vi "GEvt-Generate State Change Log.vi"(0 "CSM Global Log Event":refnum<user-event>, 1 "Current State":string, 2 "Arguments":string, 3 "Source Message.*State":string, 4 "Source Message.*Arguments":string, 5 "Source Module":string, 6 "Name(\"\" to use uuid)":string, 10 "CSM:LogFilter.lvclass":refnum<class "LogFilter.lvclass">) -> (14 "CSM Global Log Event out":refnum<user-event>, 16 "event data":T1={"Name(\"\" to use uuid)"="", "Current State"="", "Arguments"="", "Source Message"={"‘State"="", "’Arguments"="", "’Error"={"status"=FALSE, "code"=0, "source"=""}}, "Source Module"="", "Complete(T)/Start(F)"=FALSE, "LogType"=enum."State Change"})   [LabVIEW 2020, in "Communicable State Machine.lvlib"]
uses:
  Communicable State Machine.lvlib
  _CSM_GlobalLog_MSG.ctl
  _CSM_Response Source Message.ctl
  _CSM_GlobalLog_MSG_TYPE.ctl
  LogFilter.lvclass
  Filter Check.vi
  Group Check - CSM.vi
  Group Check - LogType.vi
  Group Check - State.vi
  CSM Check - LogType.vi
  CSM Check - State.vi
  CSM Check - StateType.vi
  Group Check - StateType.vi
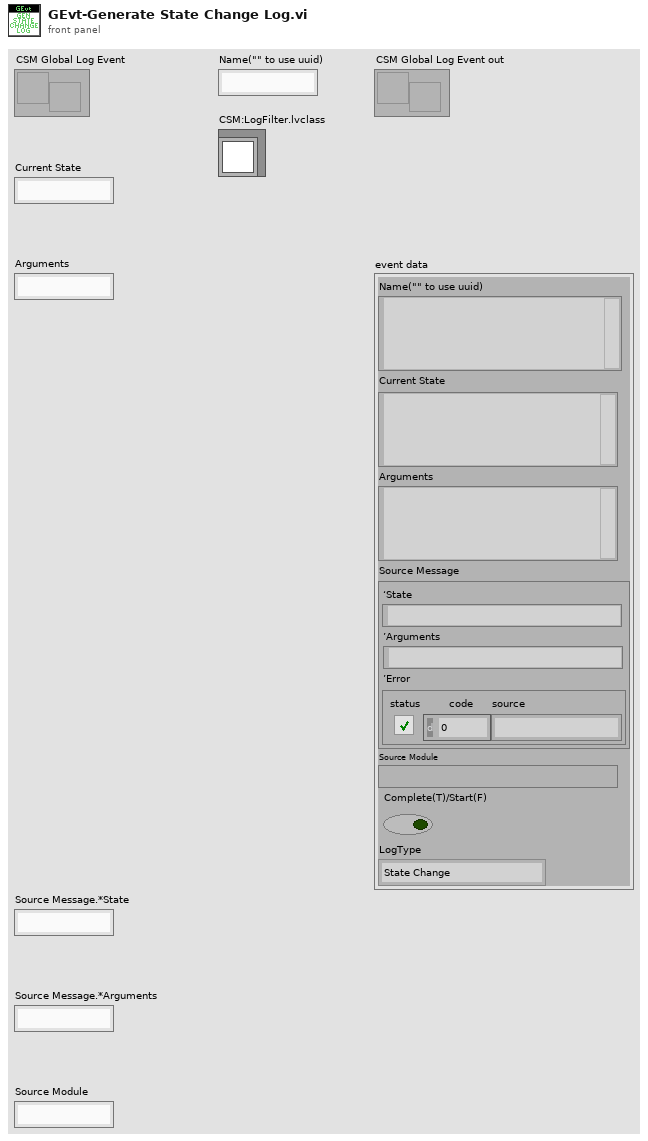
[diagram p1: front panel]
types:
  T1 = typedef "Communicable State Machine.lvlib/_CSM_GlobalLog_MSG.ctl" = cluster{"Name(\"\" to use uuid)":string, "Current State":string, "Arguments":string, "Source Message":T2, "Source Module":string, "Complete(T)/Start(F)":bool, "LogType":T3}
  T2 = typedef "Communicable State Machine.lvlib/_CSM_Response Source Message.ctl" = cluster{"‘State":string, "’Arguments":string, "’Error":errorcluster}
  T3 = typedef "Communicable State Machine.lvlib/_CSM_GlobalLog_MSG_TYPE.ctl" = enum16{"User Log", "State Change", "Status", "Interrupt", "Register", "Unregister", "Error Log", "Module Created", "Module Destroyed"}
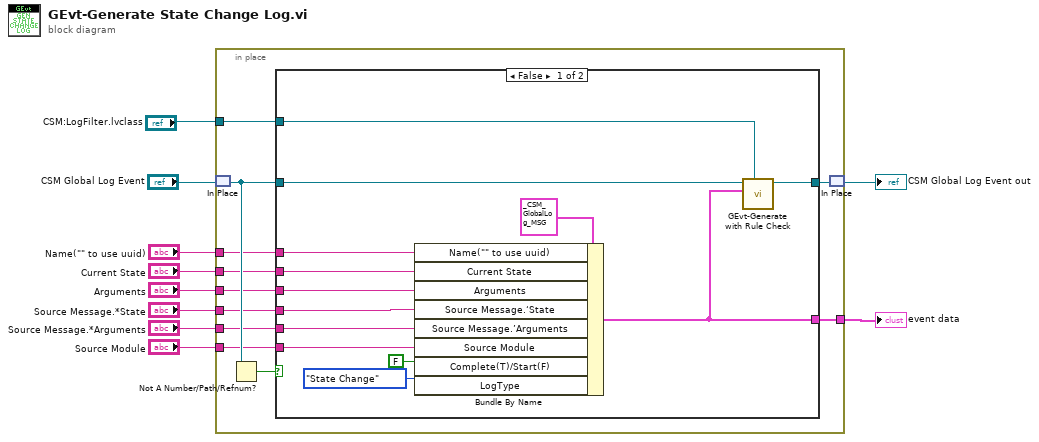
[diagram p0: block diagram]
diagram:
  n1 = in-place {
    in-place-border: [w18] -> w8
    in-place-border: "Name(\"\" to use uuid)" -> [w17]
    in-place-border: "Current State" -> [w16]
    in-place-border: "Arguments" -> [w15]
    in-place-border: "Source Message.*State" -> [w14]
    in-place-border: "Source Message.*Arguments" -> [w13]
    in-place-border: "Source Module" -> [w12]
    in-place-border: "CSM:LogFilter.lvclass" -> [w11]
    n2 = in-place-match #1("CSM Global Log Event") -> (w20:refnum<user-event>)
    n3 = Not A Number/Path/Refnum?(number/path/refnum=w20) -> (NaN/Path/Refnum?=w21:bool)
    n4 = case shown="False" w21 {
      tunnel: w20 -> [w34 w35]
      tunnel: [w33 w35] -> w19
      tunnel: [w22 _] -> w18
      tunnel: w17 -> [w29 _]
      tunnel: w16 -> [w28 _]
      tunnel: w15 -> [w27 _]
      tunnel: w14 -> [w26 _]
      tunnel: w13 -> [w25 _]
      tunnel: w12 -> [w24 _]
      tunnel: w11 -> [w23 _]
      frame False {
        n5 = Bundle By Name(cluster=T1 {"Name(\"\" to use uuid)"="", "Current State"="", "Arguments"="", "Source Message"={"‘State"="", "’Arguments"="", "’Error"={"status"=FALSE, "code"=0, "source"=""}}, "Source Module"="", "Complete(T)/Start(F)"=FALSE, "LogType"=enum."State Change"} ("event data"), "Name(\"\" to use uuid)"=w29, "Current State"=w28, "Arguments"=w27, "Source Message.‘State"=w26, "Source Message.’Arguments"=w25, "Source Module"=w24, "Complete(T)/Start(F)"=FALSE, "LogType"=_CSM_GlobalLog_MSG_TYPE."State Change" ("Type")) -> (w22:T1)
        n6 = call "GEvt-Generate with Rule Check.vi"("LogFilter in"=w23, "event data"=w22, "CSM Global Log Event in"=w34) -> ("CSM Global Log Event out"=w33:refnum<user-event>)  [unwired: 8 in]
      }
      frame True {
      }
    }
    n7 = in-place-match #1(w19) -> (→"CSM Global Log Event out":refnum<user-event>)
  }
  "event data" <- w8
